vi "sever-client.vi"() -> ()   [LabVIEW 2020]
uses:
  <vilib>/Utility/sysdir.llb/System Directory Type.ctl
panel:
  in  "s 6":bool=TRUE
  in  "s 5":bool
  in  "s 4":bool=TRUE
  in  "批量发送菜单":bool
  out "接收数据":string
  in  "发送数据":string
  out "远程端口":u16
  out "远程地址":string
  in  "批量发送":string[][](table)=[["Date", "Delay(ms)"], ["", ""], ["", ""], ["", ""], ["", ""], ["", ""]]
  in  "定时间隔毫秒":dbl=1000.0
  in  "定时发送":bool
  out "当前发送":string
  out "数值":dbl
  out "times":dbl
  in  "s 3":bool
  out "添加的路径":path
  out "每小时读码次数":dbl
  in  "s 2":bool
  out "时间统计":string
  in  "s":bool
  out "total times":dbl
  out "standard output":string caption="PING标准输出"
  in  "停止":bool
  in  "开启检测模式":bool
  out "误码次数":dbl
  in  "标准码词":string="\r"
  in  "十六进制显示":bool
  in  "自动换行":bool=TRUE
  in  "时间显示":bool=TRUE
  in  "接收超时毫秒":i32=200
  in  "清空接收数据区":bool
  in  "读取的字节":i32=500
  in  "十六进制发送":bool=TRUE
  in  "清空发送数据区":bool
  in  "发送超时毫秒":i32=200
  in  "发送":bool
  in  "数据保存":bool
  in  "路径":path
  in  "服务器IP地址":string="192.168.1.103"
  in  "sever-client":u16(ring) items=["TCP-Sever", "TCP-client"]
  in  "服务器端口号":u16=34567
  in  "开始":bool
  out "错误输出":errorcluster caption="TCP错误输出"
  # "V1.0.1"
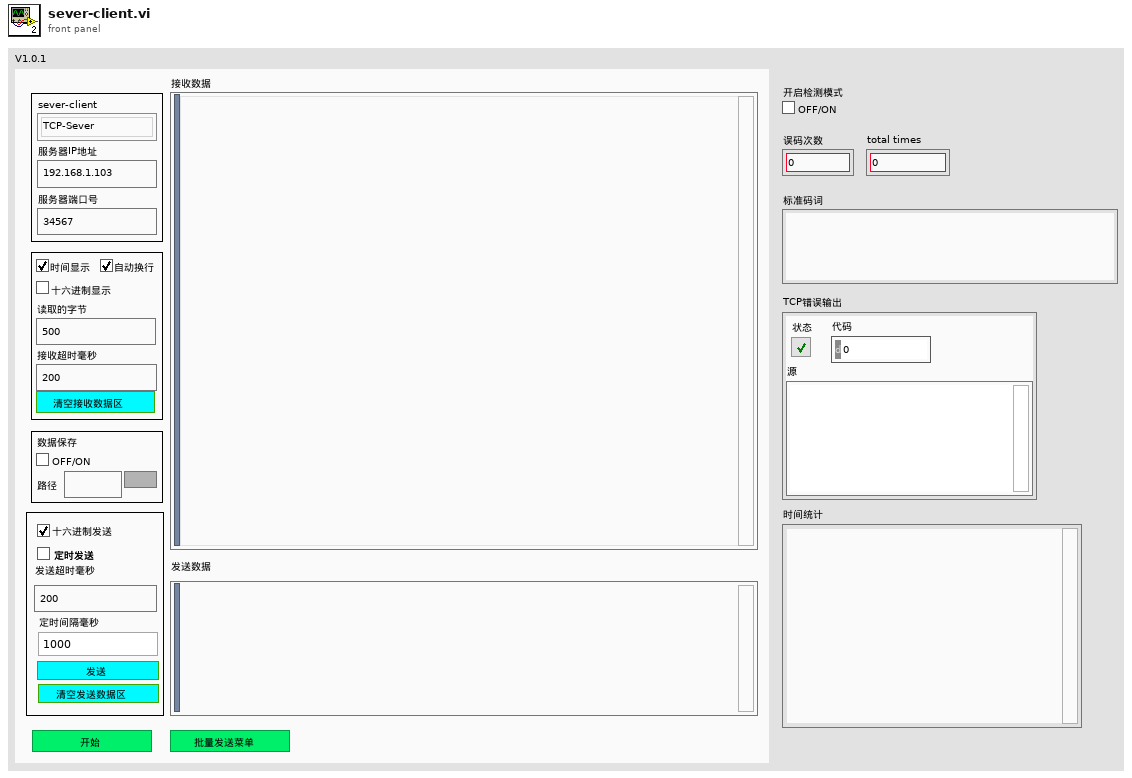
[diagram p1: front panel]
types:
  T1 = typedef "System Directory Type.ctl" = i32
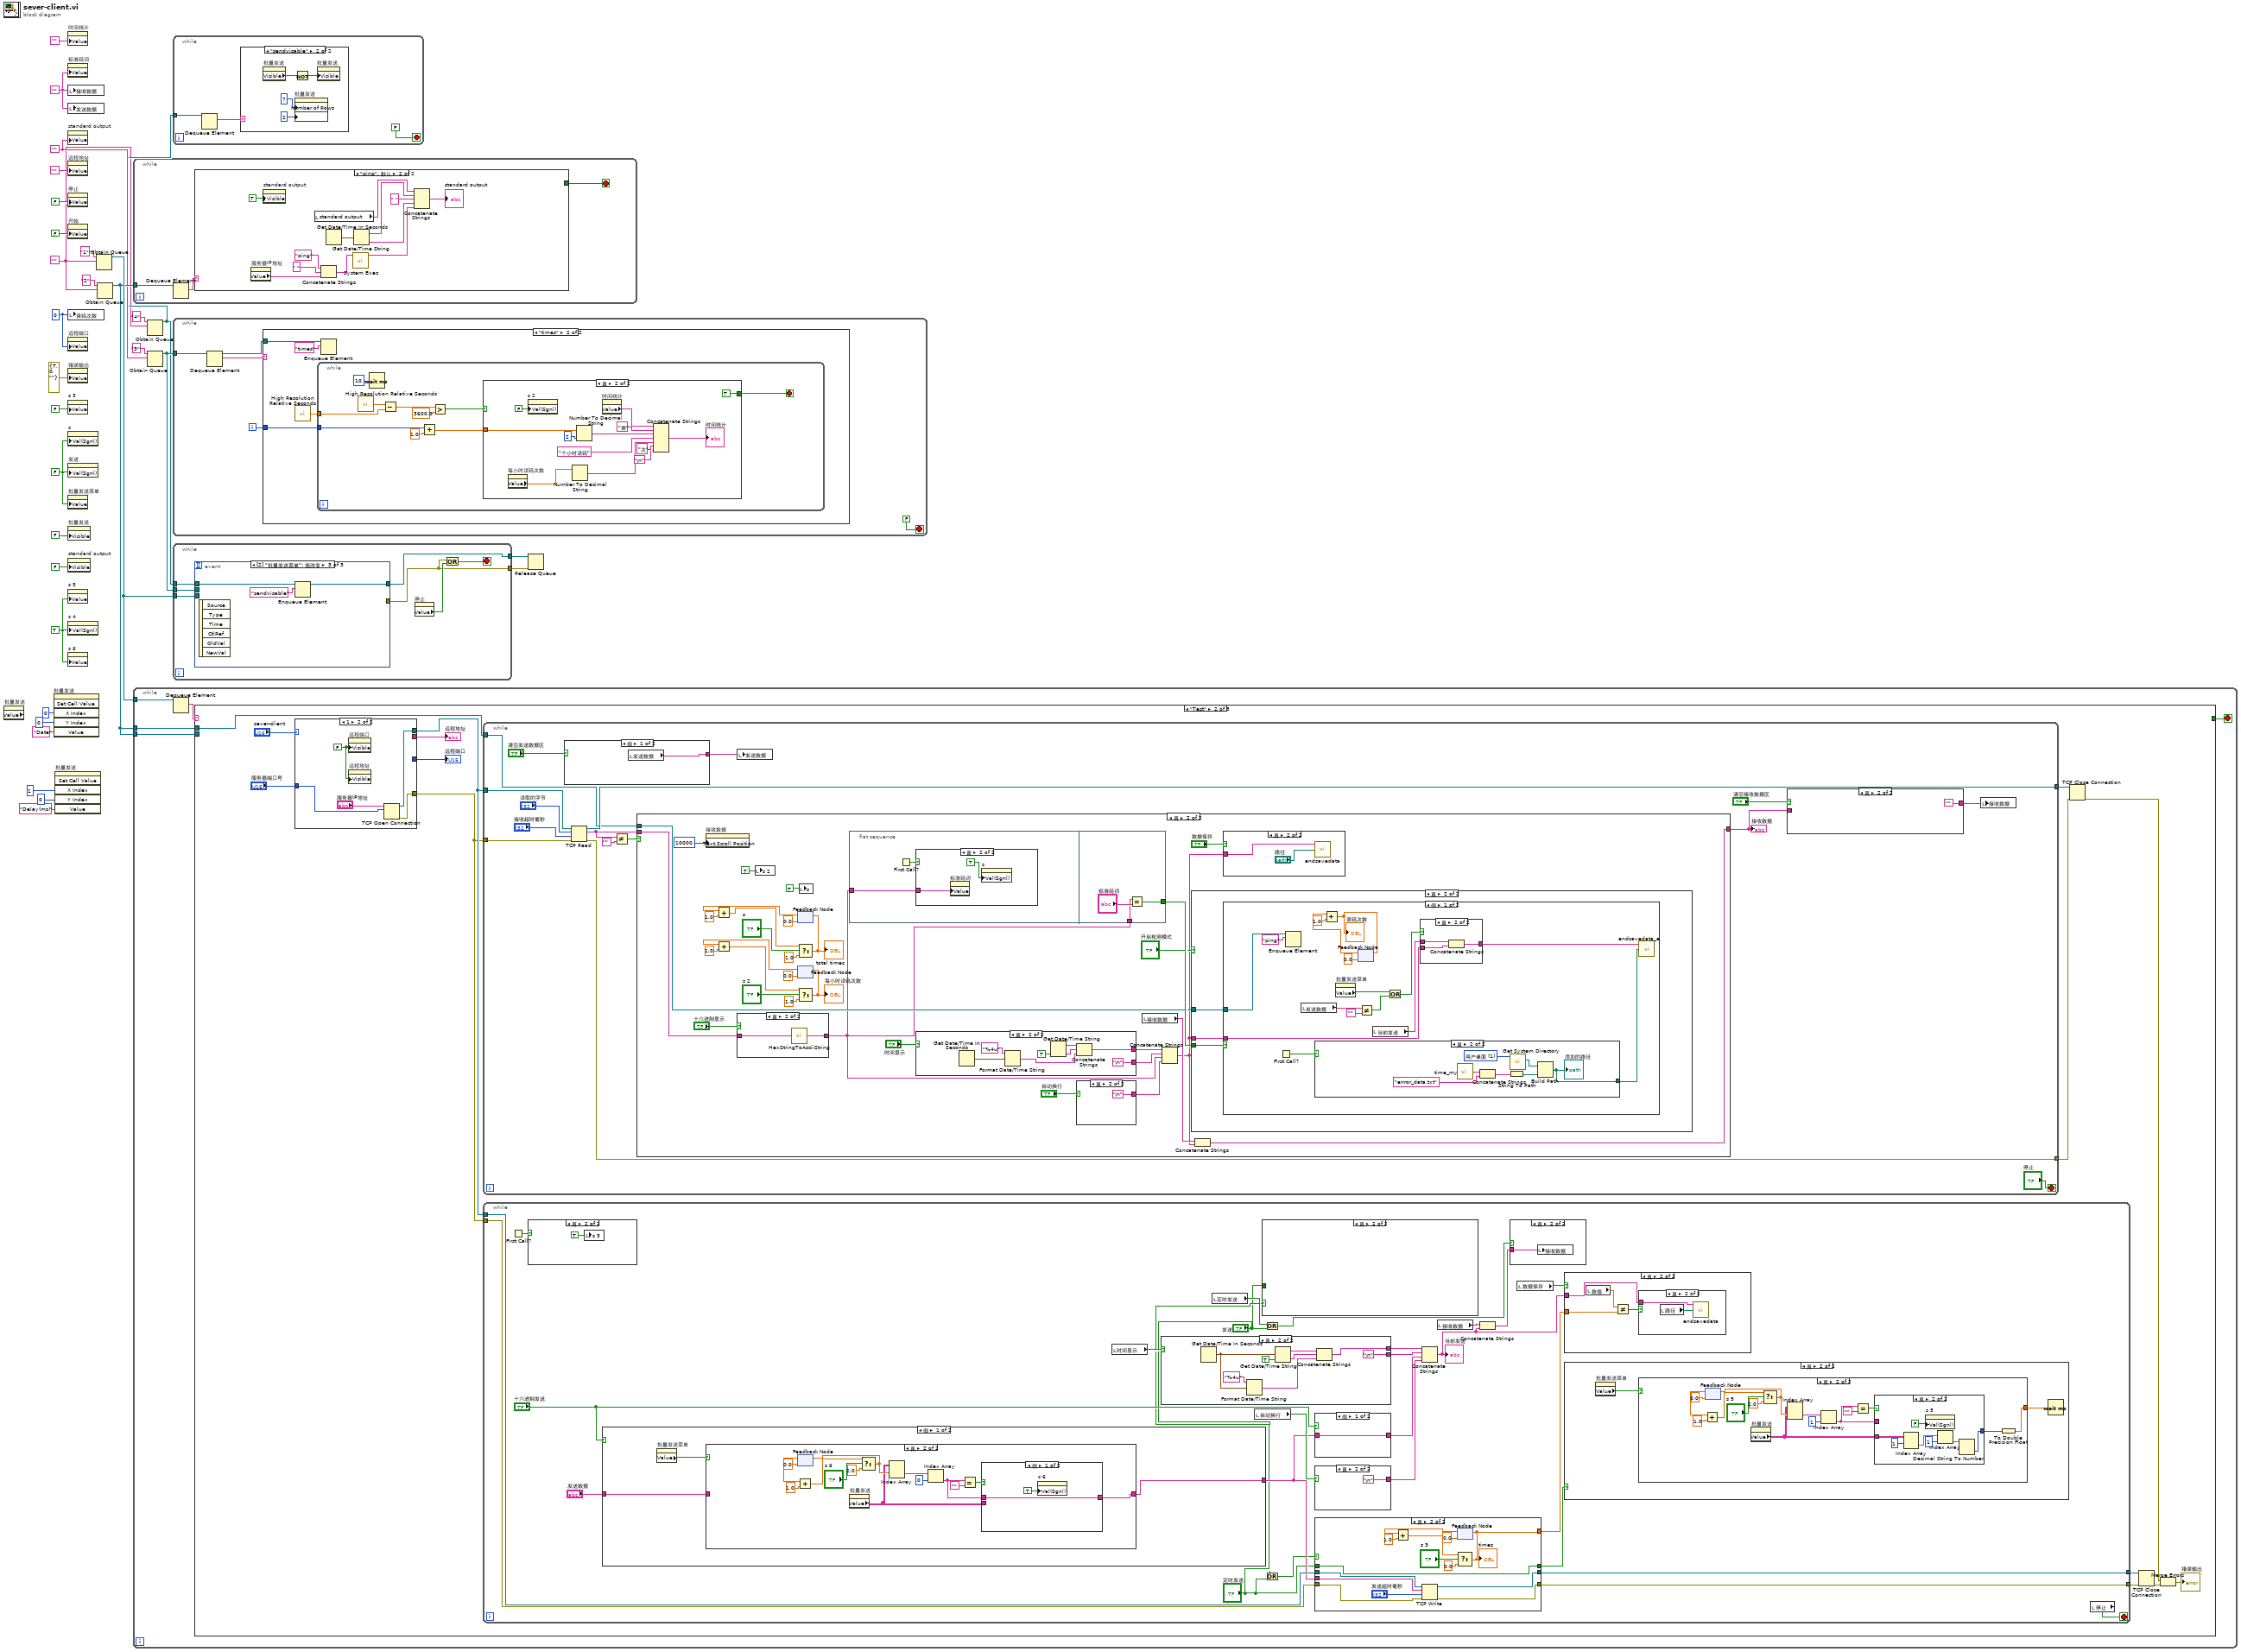
[diagram p0: block diagram]
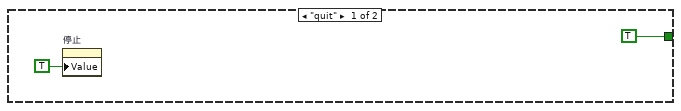
[diagram p5: hidden frame]
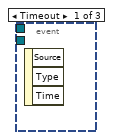
[diagram p6: hidden frame]
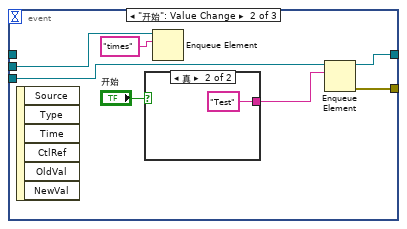
[diagram p7: hidden frame]
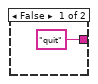
[diagram p8: hidden frame]
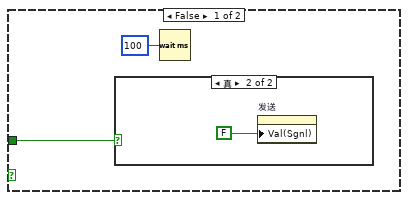
[diagram p10: hidden frame]
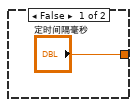
[diagram p13: hidden frame]
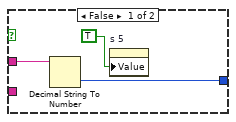
[diagram p14: hidden frame]
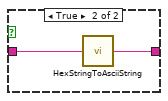
[diagram p17: hidden frame]
diagram:
  w8 = TRUE ("值(信号)")
  w7 = u16 0 ("远程端口")
  w15 = ""
  w10 = FALSE ("值(信号)")
  w18 = ""
  w12 = ""
  n1 = property on="批量发送" class="Tbl (严格)" props=["Value"]() -> ()  [unwired: 2 in, 3 out]
  n2 = invoke on="批量发送" class="Tbl (严格)" method="Set Cell Value"("X Index"=0 ("X索引"), "Y Index"=0 ("Y索引"), "Value"="Date" ("值")) -> ()  [unwired: 3 in, 6 out]
  n3 = invoke on="批量发送" class="Tbl (严格)" method="Set Cell Value"("X Index"=1 ("X索引"), "Y Index"=0 ("Y索引"), "Value"="Delay(ms)" ("值")) -> ()  [unwired: 3 in, 6 out]
  n4 = property on="时间统计" class="Str"("Value"="") -> ()  [unwired: 2 in, 2 out]
  n5 = property on="标准码词" class="Str"("Value"=w15) -> ()  [unwired: 2 in, 2 out]
  n6 = local write "接收数据"(w15) -> ()
  n7 = local write "发送数据"(w15) -> ()
  n8 = property on="standard output" class="Str"("Value"=w18) -> ()  [unwired: 2 in, 2 out]
  n9 = property on="远程地址" class="Str"("Value"="") -> ()  [unwired: 2 in, 2 out]
  n10 = property on="停止" class="Bool (严格)"("Value"=FALSE ("停止")) -> ()  [unwired: 2 in, 2 out]
  n11 = property on="开始" class="Bool (严格)"("Value"=FALSE ("开始")) -> ()  [unwired: 2 in, 2 out]
  n12 = local write "误码次数"(w7) -> ()
  n13 = property on="远程端口" class="DigNum (严格)"("Value"=w7) -> ()  [unwired: 2 in, 2 out]
  n14 = property on="错误输出" class="Clust (严格)"("Value"=errorcluster {"status"=TRUE, "code"=0, "source"=""} ("错误输出")) -> ()  [unwired: 2 in, 2 out]
  n15 = property on="s 3" class="Bool (严格)"("Value"=FALSE ("s 3")) -> ()  [unwired: 2 in, 2 out]
  n16 = property on="s" class="Bool (严格)"("Val(Sgnl)"=w10) -> ()  [unwired: 2 in, 2 out]
  n17 = property on="发送" class="Bool (严格)"("Val(Sgnl)"=w10) -> ()  [unwired: 2 in, 2 out]
  n18 = property on="批量发送菜单" class="Bool (严格)"("Value"=w10) -> ()  [unwired: 2 in, 2 out]
  n19 = property on="批量发送" class="Tbl (严格)"("Visible"=FALSE ("可见")) -> ()  [unwired: 2 in, 2 out]
  n20 = property on="standard output" class="Str"("Visible"=FALSE ("可见")) -> ()  [unwired: 2 in, 2 out]
  n21 = property on="s 5" class="Bool (严格)"("Value"=w8) -> ()  [unwired: 2 in, 2 out]
  n22 = property on="s 4" class="Bool (严格)"("Val(Sgnl)"=w8) -> ()  [unwired: 2 in, 2 out]
  n23 = property on="s 6" class="Bool (严格)"("Value"=w8) -> ()  [unwired: 2 in, 2 out]
  n24 = Obtain Queue(name (unnamed)="1" ("名称（未命名）"), element data type=w12) -> (queue out=w29:refnum<queue>)  [unwired: 3 in, 2 out]
  n25 = Obtain Queue(name (unnamed)="2" ("名称（未命名）"), element data type=w12) -> (queue out=w25:refnum<queue>)  [unwired: 3 in, 2 out]
  n26 = while {
    tunnel: w25 -> [w31]
    stop <- w32 stop-if-true
    n27 = Dequeue Element(queue=w31) -> (element=w33:string)  [unwired: 2 in, 3 out]
    n28 = case shown="\"ping\", 默认" w33 {
      tunnel: [TRUE _] -> w32
      frame "quit" {
        n29 = property on="停止" class="Bool (严格)"("Value"=TRUE ("停止")) -> ()  [unwired: 2 in, 2 out]
      }
      frame "ping", Default {
        n30 = property on="服务器IP地址" class="Str"() -> ("Value"=w45:string)  [unwired: 2 in, 2 out]
        n31 = property on="standard output" class="Str"("Visible"=TRUE ("可见")) -> ()  [unwired: 2 in, 2 out]
        n32 = local read "standard output"() -> (w37:string)
        n33 = Concatenate Strings("ping" ("字符串"), " " ("字符串"), w45) -> (w44:string)
        n34 = Get Date/Time In Seconds() -> (seconds since 1Jan1904=w42:timestamp)
        n35 = call <vilib>:"System Exec.vi"("command line"=w44) -> ("standard output"=w43:string)  [unwired: 7 in, 3 out]
        n36 = Get Date/Time String(seconds (now)=w42) -> (date string=w41:string, time string=w39:string)  [unwired: 2 in]
        n37 = Concatenate Strings(w37, w41, " " ("字符串"), w39, w43) -> (→"standard output":string)
      }
    }
  }
  n38 = while {
    tunnel: w29 -> [w50]
    tunnel: w25 -> [w49]
    tunnel: w25 -> [w48]
    stop <- w52 stop-if-true
    n39 = Dequeue Element(queue=w50) -> (element=w51:string)  [unwired: 2 in, 3 out]
    n40 = case shown="\"Test\"" w51 {
      tunnel: [_ _ TRUE] -> w52
      tunnel: w49 -> [_ w61 _]
      tunnel: w48 -> [_ _ w342]
      frame "假", Default {
      }
      frame "Test" {
        n41 = case shown="1" "sever-client" {
          tunnel: "服务器端口号" -> [w226 w231]
          tunnel: [w225 w230] -> w60
          tunnel: [w224 w229] -> w59
          tunnel: [w223 _] -> w64
          tunnel: [w222 _] -> w63
          frame 0, Default {
            w221 = TRUE
            n42 = property on="远程端口" class="DigNum (严格)"("Visible"=w221) -> ()  [unwired: 2 in, 2 out]
            n43 = property on="远程地址" class="Str"("Visible"=w221) -> ()  [unwired: 2 in, 2 out]
            n44 = call <vilib>:"TCP Listen.vi"("port"=w226) -> ("error out"=w224:errorcluster, "remote port"=w222:u16, "remote address"=w223:string, "connection ID"=w225:refnum<k5>)  [unwired: 6 in, 1 out]
          }
          frame 1 {
            w227 = FALSE
            n45 = property on="远程端口" class="DigNum (严格)"("Visible"=w227) -> ()  [unwired: 2 in, 2 out]
            n46 = property on="远程地址" class="Str"("Visible"=w227) -> ()  [unwired: 2 in, 2 out]
            n47 = TCP Open Connection(address="服务器IP地址", remote port or service name=w231) -> (connection ID=w230:refnum<k5>, error out=w229:errorcluster)  [unwired: 3 in]
          }
        }
        "远程地址" <- w64
        "远程端口" <- w63
        n48 = while {
          tunnel: [w245] -> w54
          tunnel: [w237] -> w62
          tunnel: w61 -> [w236]
          tunnel: w60 -> [w234]
          tunnel: w59 -> [w233]
          stop <- "停止" stop-if-true
          n49 = case shown="假" "清空发送数据区" {
            tunnel: [w248 ""] -> w238
            frame False {
              n50 = local read "发送数据"() -> (w248:string)
            }
            frame True {
            }
          }
          n51 = TCP Read(connection ID=w234, bytes to read="读取的字节", error in (no error)=w233, 9:"接收超时毫秒") -> (connection ID out=w245:refnum<k5>, data out=w243:string, error out=w237:errorcluster)  [unwired: 1 in]
          n52 = Not Equal?(x=w243, y="") -> (x != y?=w232:bool)
          n53 = case shown="真" w232 {
            tunnel: w243 -> [_ w284]
            tunnel: [w257 w286] -> w240
            tunnel: w236 -> [_ w280]
            frame False {
              n54 = local read "接收数据"() -> (w257:string)
            }
            frame True {
              n55 = property on="接收数据" class="Str"("Text.Scroll Position"=u32 10000 ("文本.滚动条位置")) -> ()  [unwired: 2 in, 2 out]
              n56 = case shown="真" "十六进制显示" {
                tunnel: [w328 w330] -> w262
                tunnel: w284 -> [w328 w329]
                frame False {
                }
                frame True {
                  n57 = call "HexStringToAsciiString.vi"("输入Hex字符串"=w329) -> ("输出Ascii"=w330:string)
                }
              }
              n58 = local write "s 2"(TRUE ("值(信号)")) -> ()
              n59 = feedback #1(0.0 ("x")) -> (w276:dbl)
              n60 = Add(x=w276, y=1.0) -> (x+y=w275:dbl)
              n61 = Select(t=w275, s="s", f=1.0) -> (s? t:f=w272:dbl)
              "total times" <- w272
              n62 = feedback-in #1(w272) -> ()
              n63 = feedback #2(0.0 ("x")) -> (w269:dbl)
              n64 = Add(x=w269, y=1.0) -> (x+y=w270:dbl)
              n65 = Select(t=w270, s="s 2", f=1.0) -> (s? t:f=w265:dbl)
              "每小时读码次数" <- w265
              n66 = feedback-in #2(w265) -> ()
              n67 = local write "s"(TRUE ("值(信号)")) -> ()
              n68 = flat-sequence {
                tunnel: w262 -> [w290]
                tunnel: w262 -> [w294]
                tunnel: [w295] -> w283
                frame #0 {
                  n69 = First Call?() -> (First Call?: T/F=w291:bool)
                  n70 = case shown="真" w291 {
                    tunnel: w290 -> [_ w293]
                    frame False {
                    }
                    frame True {
                      n71 = property on="标准码词" class="Str"("Value"=w293) -> ()  [unwired: 2 in, 2 out]
                      n72 = property on="s" class="Bool (严格)"("Val(Sgnl)"=TRUE ("值(信号)")) -> ()  [unwired: 2 in, 2 out]
                    }
                  }
                }
                frame #1 {
                  n73 = Equal?(x=w294, y="标准码词") -> (x = y?=w295:bool)
                }
              }
              n74 = case shown="真" "时间显示" {
                tunnel: [_ w338] -> w264
                tunnel: [_ "\n"] -> w263
                frame False {
                }
                frame True {
                  n75 = Get Date/Time In Seconds() -> (seconds since 1Jan1904=w335:timestamp)
                  n76 = Format Date/Time String(time format string (%c)="%4u" ("时间格式字符串(%c)"), seconds (now)=w335) -> (date/time string=w334:string)  [unwired: 1 in]
                  n77 = Get Date/Time String(want seconds? (F)=TRUE ("需要秒？(F)")) -> (date string=w340:string, time string=w339:string)  [unwired: 2 in]
                  n78 = Concatenate Strings(w340, w339, w334) -> (w338:string)
                }
              }
              n79 = case shown="真" "自动换行" {
                tunnel: [_ "\n"] -> w261
                frame False {
                }
                frame True {
                }
              }
              n80 = local read "接收数据"() -> (w288:string)
              n81 = Concatenate Strings(w264, w263, w262, w261) -> (w260:string)
              n82 = case shown="真" "开启检测模式" {
                tunnel: w283 -> [_ w299]
                tunnel: w280 -> [_ w298]
                tunnel: w260 -> [_ w297]
                frame False {
                }
                frame True {
                  n83 = case shown="假" w299 {
                    tunnel: w298 -> [w310 _]
                    tunnel: w297 -> [w306 _]
                    frame False {
                      n84 = First Call?() -> (First Call?: T/F=w309:bool)
                      n85 = Enqueue Element(queue=w310, element="ping" ("元素")) -> ()  [unwired: 2 in, 3 out]
                      n86 = local read "发送数据"() -> (w304:string)
                      n87 = case shown="真" w309 {
                        tunnel: [w320 w323] -> w308
                        frame False {
                          n88 = local read "添加的路径"() -> (w320:path)
                        }
                        frame True {
                          w327 = T1 1 items=["用户目录"=0, "用户桌面"=1, "用户文档"=2, "用户应用程序数据"=3, "用户设置"=4, "用户临时目录"=5, "公共文档"=6, "公共应用程序数据"=7, "公共设置"=8, "公共缓存"=13, "系统核心库"=9, "系统安装库"=10, "应用程序文件"=11, "启动盘根目录"=12] ("system directory type")
                          n89 = call "time_my.vi"() -> ("时间"=w321:string)
                          n90 = Concatenate Strings(w321, "errror_data.txt") -> (w325:string)
                          n91 = String To Path(string=w325) -> (path=w324:path)
                          n92 = call <vilib>:"Get System Directory.vi"("system directory type"=w327) -> ("system directory"=w326:path)  [unwired: 10 in]
                          n93 = Build Path(base path=w326, name or relative path=w324) -> (appended path=w323:path)
                          "添加的路径" <- w323
                        }
                      }
                      n94 = property on="批量发送菜单" class="Bool (严格)"() -> ("Value"=w302:bool)  [unwired: 2 in, 2 out]
                      n95 = feedback #3(0.0) -> (w312:dbl)
                      n96 = Add(x=w312, y=1.0) -> (x+y=w314:dbl)
                      "误码次数" <- w314
                      n97 = feedback-in #3(w314) -> ()
                      n98 = Not Equal?(x=w304, y="") -> (x != y?=w303:bool)
                      n99 = local read "当前发送"() -> (w305:string)
                      n100 = Or(x=w302, y=w303) -> (x .or. y?=w301:bool)
                      n101 = case shown="真" w301 {
                        tunnel: [w316 w317] -> w307
                        tunnel: w306 -> [w316 w318]
                        tunnel: w305 -> [_ w319]
                        frame False {
                        }
                        frame True {
                          n102 = Concatenate Strings(w319, w318) -> (w317:string)
                        }
                      }
                      n103 = call "endsavedata_e.vi"("文件路径（使用对话框）"=w308, "文本"=w307) -> ()  [unwired: 1 in, 2 out]
                    }
                    frame True {
                    }
                  }
                }
              }
              n104 = Concatenate Strings(w288, w260) -> (w286:string)
              n105 = case shown="真" "数据保存" {
                tunnel: w260 -> [_ w331]
                frame False {
                }
                frame True {
                  n106 = call "endsavedata.vi"("文件路径（使用对话框）"="路径", "文本"=w331) -> ()  [unwired: 1 in, 2 out]
                }
              }
            }
          }
          "接收数据" <- w240
          n107 = local write "发送数据"(w238) -> ()
          n108 = case shown="真" "清空接收数据区" {
            tunnel: [w253 ""] -> w242
            tunnel: w240 -> [w251 _]
            frame False {
              n109 = String Length(string=w251) -> (length=w255:i32)
              n110 = Greater?(x=w255, y=10000) -> (0:w254:bool)
              n111 = Select(t="", s=w254, f=w251) -> (s? t:f=w253:string)
            }
            frame True {
            }
          }
          n112 = local write "接收数据"(w242) -> ()
        }
        n113 = while {
          tunnel: w60 -> [w92]
          tunnel: w59 -> [w91]
          tunnel: [w90] -> w58
          tunnel: [w73] -> w53
          stop <- w89 stop-if-true
          n114 = First Call?() -> (First Call?: T/F=w77:bool)
          n115 = case shown="真" w77 {
            frame False {
            }
            frame True {
              n116 = local write "s 3"(TRUE ("s 3")) -> ()
            }
          }
          n117 = case shown="假" "十六进制发送" {
            selector: "十六进制发送" -> [_ w181]
            tunnel: "发送数据" -> [w157 w184]
            tunnel: [w156 w183] -> w82
            frame False {
              n118 = property on="批量发送菜单" class="Bool (严格)"() -> ("Value"=w155:bool)  [unwired: 2 in, 2 out]
              n119 = case shown="真" w155 {
                tunnel: [w158 w161] -> w156
                tunnel: w157 -> [w158 _]
                frame False {
                }
                frame True {
                  n120 = feedback #4(0.0 ("x")) -> (w169:dbl)
                  n121 = Add(x=w169, y=1.0) -> (x+y=w166:dbl)
                  n122 = property on="批量发送" class="Tbl (严格)"() -> ("Value"=w159:string[][])  [unwired: 2 in, 2 out]
                  n123 = Select(t=w166, s="s 6", f=2.0) -> (s? t:f=w165:dbl)
                  n124 = feedback-in #4(w165) -> ()
                  n125 = Index Array(array=w159, index (row)=w165) -> (element=w172:string[])  [unwired: 1 in]
                  n126 = Index Array(array=w172, index=0 ("索引")) -> (element=w160:string)
                  n127 = Equal?(x=w160, y="") -> (x = y?=w162:bool)
                  n128 = case shown="假" w162 {
                    tunnel: [w174 w178] -> w161
                    tunnel: w160 -> [w174 _]
                    tunnel: w159 -> [_ w180]
                    frame False {
                      n129 = property on="s 6" class="Bool (严格)"("Val(Sgnl)"=TRUE ("值(信号)")) -> ()  [unwired: 2 in, 2 out]
                    }
                    frame True {
                      n130 = Index Array(array=w180, index (row)=1 ("索引 (行)")) -> (element=w179:string[])  [unwired: 1 in]
                      n131 = property on="s 6" class="Bool (严格)"("Val(Sgnl)"=FALSE ("值(信号)")) -> ()  [unwired: 2 in, 2 out]
                      n132 = Index Array(array=w179, index=0 ("索引")) -> (element=w178:string)
                    }
                  }
                }
              }
            }
            frame True {
              n133 = local read "times"() -> (→"数值":dbl)
              n134 = case shown="真" "批量发送菜单" {
                tunnel: w184 -> [w187 _]
                tunnel: [w186 w198] -> w183
                tunnel: w181 -> [_ w197]
                frame False {
                  n135 = call "AsciiStringToHexString.vi"("输入Asciistring1"=w187) -> ("输出HexString"=w186:string)
                }
                frame True {
                  n136 = feedback #5(0.0 ("x")) -> (w200:dbl)
                  n137 = Add(x=w200, y=1.0) -> (x+y=w195:dbl)
                  n138 = Select(t=w195, s="s 4", f=2.0) -> (s? t:f=w194:dbl)
                  n139 = feedback-in #5(w194) -> ()
                  n140 = Index Array(array="批量发送", index (row)=w194) -> (element=w203:string[])  [unwired: 1 in]
                  n141 = Index Array(array=w203, index=0 ("索引")) -> (element=w189:string)
                  n142 = Equal?(x=w189, y="") -> (x = y?=w191:bool)
                  n143 = case shown="假" w191 {
                    tunnel: [w205 w209] -> w190
                    tunnel: w189 -> [w205 _]
                    tunnel: "批量发送" -> [_ w211]
                    frame False {
                      n144 = property on="s 4" class="Bool (严格)"("Val(Sgnl)"=TRUE ("值(信号)")) -> ()  [unwired: 2 in, 2 out]
                    }
                    frame True {
                      n145 = Index Array(array=w211, index (row)=1 ("索引 (行)")) -> (element=w210:string[])  [unwired: 1 in]
                      n146 = property on="s 4" class="Bool (严格)"("Val(Sgnl)"=FALSE ("值(信号)")) -> ()  [unwired: 2 in, 2 out]
                      n147 = Index Array(array=w210, index=0 ("索引")) -> (element=w209:string)
                    }
                  }
                  n148 = case shown="真" w197 {
                    tunnel: [w212 w214] -> w198
                    tunnel: w190 -> [w212 w213]
                    frame False {
                    }
                    frame True {
                      n149 = call "AsciiStringToHexString.vi"("输入Asciistring1"=w213) -> ("输出HexString"=w214:string)
                    }
                  }
                }
              }
            }
          }
          n150 = local read "时间显示"() -> (w74:bool)
          n151 = case shown="真" w74 {
            tunnel: [_ w135] -> w86
            tunnel: [_ "\n"] -> w85
            frame False {
            }
            frame True {
              n152 = Get Date/Time In Seconds() -> (seconds since 1Jan1904=w131:timestamp)
              n153 = Format Date/Time String(time format string (%c)="%4u" ("时间格式字符串(%c)"), seconds (now)=w131) -> (date/time string=w132:string)  [unwired: 1 in]
              n154 = Get Date/Time String(seconds (now)=w131, want seconds? (F)=TRUE ("需要秒？(F)")) -> (date string=w136:string, time string=w133:string)  [unwired: 1 in]
              n155 = Concatenate Strings(w136, w133, w132) -> (w135:string)
            }
          }
          n156 = local read "定时发送"() -> (w72:bool)
          n157 = local read "自动换行"() -> (w87:bool)
          n158 = case shown="真" "定时发送" {
            tunnel: "发送" -> [w94 _]
            frame False {
              n159 = case shown="真" w94 {
                frame False {
                }
                frame True {
                  n160 = property on="发送" class="Bool (严格)"("Val(Sgnl)"=FALSE ("值(信号)")) -> ()  [unwired: 2 in, 2 out]
                }
              }
              n161 = Wait (ms)(milliseconds to wait=u32 100 ("等待时间（毫秒）")) -> ()  [unwired: 1 out]
            }
            frame True {
            }
          }
          n162 = Or(x=w72, y="发送") -> (x .or. y?=w71:bool)
          n163 = Or(x="发送", y="定时发送") -> (x .or. y?=w70:bool)
          n164 = case shown="假" "十六进制发送" {
            tunnel: [w126 w128] -> w81
            tunnel: w82 -> [w126 w127]
            frame False {
            }
            frame True {
              n165 = call "HexStringToAsciiString.vi"("输入Hex字符串"=w127) -> ("输出Ascii"=w128:string)
            }
          }
          n166 = case shown="真" w87 {
            tunnel: [_ "\n"] -> w83
            frame False {
            }
            frame True {
            }
          }
          n167 = case shown="真" w70 {
            tunnel: w82 -> [_ w150]
            tunnel: [w140 w154] -> w73
            tunnel: [w139 w153] -> w90
            tunnel: w92 -> [w140 w152]
            tunnel: w91 -> [w139 w151]
            tunnel: [_ w143] -> w76
            tunnel: "定时发送" -> [w138 w142]
            tunnel: [w138 w142] -> w69
            frame False {
            }
            frame True {
              n168 = TCP Write(connection ID=w152, data in=w150, error in (no error)=w151, 9:"发送超时毫秒") -> (connection ID out=w154:refnum<k5>, error out=w153:errorcluster)  [unwired: 1 out]
              n169 = feedback #6(0.0 ("x")) -> (w144:dbl)
              n170 = Add(x=w144, y=1.0) -> (x+y=w149:dbl)
              n171 = Select(t=w149, s="s 3", f=0.0) -> (s? t:f=w143:dbl)
              "times" <- w143
              n172 = feedback-in #6(w143) -> ()
            }
          }
          n173 = Concatenate Strings(w86, w85, w81, w83) -> (w79:string)
          "当前发送" <- w79
          n174 = local read "接收数据"() -> (w84:string)
          n175 = Concatenate Strings(w84, w79) -> (w78:string)
          n176 = case shown="真" w71 {
            tunnel: w78 -> [_ w125]
            frame False {
            }
            frame True {
              n177 = local write "接收数据"(w125) -> ()
            }
          }
          n178 = local read "数据保存"() -> (w75:bool)
          n179 = case shown="真" w75 {
            tunnel: w79 -> [_ w218]
            tunnel: w76 -> [_ w216]
            frame False {
            }
            frame True {
              n180 = local read "数值"() -> (w215:dbl)
              n181 = Not Equal?(x=w215, y=w216) -> (x != y?=w217:bool)
              n182 = case shown="真" w217 {
                tunnel: w218 -> [_ w219]
                frame False {
                }
                frame True {
                  n183 = local read "路径"() -> (w220:path)
                  n184 = call "endsavedata.vi"("文件路径（使用对话框）"=w220, "文本"=w219) -> ()  [unwired: 1 in, 2 out]
                }
              }
            }
          }
          n185 = case shown="真" w69 {
            frame False {
            }
            frame True {
              n186 = property on="批量发送菜单" class="Bool (严格)"() -> ("Value"=w96:bool)  [unwired: 2 in, 2 out]
              n187 = case shown="真" w96 {
                tunnel: ["定时间隔毫秒" w99] -> w97
                frame False {
                }
                frame True {
                  n188 = feedback #7(0.0 ("x")) -> (w109:dbl)
                  n189 = Add(x=w109, y=1.0) -> (x+y=w108:dbl)
                  n190 = property on="批量发送" class="Tbl (严格)"() -> ("Value"=w103:string[][])  [unwired: 2 in, 2 out]
                  n191 = Select(t=w108, s="s 5", f=2.0) -> (s? t:f=w104:dbl)
                  n192 = feedback-in #7(w104) -> ()
                  n193 = Index Array(array=w103, index (row)=w104) -> (element=w113:string[])  [unwired: 1 in]
                  n194 = Index Array(array=w113, index=1 ("索引")) -> (element=w107:string)
                  n195 = Equal?(x=w107, y="") -> (x = y?=w105:bool)
                  n196 = case shown="真" w105 {
                    tunnel: w107 -> [w116 _]
                    tunnel: [w115 w118] -> w100
                    tunnel: w103 -> [_ w122]
                    frame False {
                      n197 = Decimal String To Number(string=w116) -> (number=w115:i32)  [unwired: 2 in, 1 out]
                      n198 = property on="s 5" class="Bool (严格)"("Value"=TRUE ("s 5")) -> ()  [unwired: 2 in, 2 out]
                    }
                    frame True {
                      n199 = Index Array(array=w122, index (row)=1 ("索引 (行)")) -> (element=w121:string[])  [unwired: 1 in]
                      n200 = property on="s 5" class="Bool (严格)"("Val(Sgnl)"=FALSE ("值(信号)")) -> ()  [unwired: 2 in, 2 out]
                      n201 = Index Array(array=w121, index=1 ("索引")) -> (element=w119:string)
                      n202 = Decimal String To Number(string=w119) -> (number=w118:i32)  [unwired: 2 in, 1 out]
                    }
                  }
                  n203 = To Double Precision Float(number=w100) -> (double precision float=w99:dbl)
                }
              }
              n204 = Wait (ms)(milliseconds to wait=w97) -> ()  [unwired: 1 out]
            }
          }
          n205 = local read "停止"() -> (w89:bool)
        }
        n206 = TCP Close Connection(connection ID=w54, error in (no error)=w62) -> (error out=w56:errorcluster)  [unwired: 1 in, 1 out]
        n207 = TCP Close Connection(connection ID=w53, error in (no error)=w58) -> (error out=w57:errorcluster)  [unwired: 1 in, 1 out]
        n208 = Merge Errors(w56, w57) -> (→"错误输出":errorcluster)
      }
      frame "quit" {
        n209 = Enqueue Element(queue=w342, element="quit" ("元素")) -> ()  [unwired: 2 in, 3 out]
      }
    }
  }
  n210 = Obtain Queue(name (unnamed)="4" ("名称（未命名）"), element data type=w12) -> (queue out=w13:refnum<queue>)  [unwired: 3 in, 2 out]
  n211 = Obtain Queue(name (unnamed)="3" ("名称（未命名）"), element data type=w18) -> (queue out=w20:refnum<queue>)  [unwired: 3 in, 2 out]
  n212 = while {
    tunnel: w13 -> [w346]
    stop <- FALSE stop-if-true
    n213 = Dequeue Element(queue=w346) -> (element=w347:string)  [unwired: 2 in, 3 out]
    n214 = case shown="\"sendvisable\"" w347 {
      frame "假", Default {
      }
      frame "sendvisable" {
        n215 = property on="批量发送" class="Tbl (严格)"() -> ("Visible"=w351:bool)  [unwired: 2 in, 2 out]
        n216 = Not(x=w351) -> (.not. x?=w350:bool)
        n217 = property on="批量发送" class="Tbl (严格)"("Number of Rows"=u32 7 ("行数"), "Number of Columns"=u32 2 ("列数")) -> ()  [unwired: 2 in, 2 out]
        n218 = property on="批量发送" class="Tbl (严格)"("Visible"=w350) -> ()  [unwired: 2 in, 2 out]
      }
    }
  }
  n219 = while {
    tunnel: w20 -> [w354]
    i -> [w353]
    stop <- FALSE stop-if-true
    n220 = Dequeue Element(queue=w354) -> (queue out=w352:refnum<queue>, element=w355:string)  [unwired: 2 in, 2 out]
    n221 = case shown="\"times\"" w355 {
      tunnel: w353 -> [_ w359]
      tunnel: w352 -> [_ w358]
      frame "假", Default {
      }
      frame "times" {
        n222 = call <vilib>:"High Resolution Relative Seconds.vi"() -> ("relative seconds"=w360:dbl)
        n223 = while {
          tunnel: w360 -> [w369]
          tunnel: w359 -> [w362]
          stop <- w365 stop-if-true
          n224 = call <vilib>:"High Resolution Relative Seconds.vi"() -> ("relative seconds"=w370:dbl)
          n225 = Wait (ms)(milliseconds to wait=u32 10 ("等待时间（毫秒）")) -> ()  [unwired: 1 out]
          n226 = Subtract(x=w370, y=w369) -> (x-y=w368:dbl)
          n227 = Add(x=w362, y=1.0) -> (x+y=w361:dbl)
          n228 = Greater?(x=w368, y=3600.0) -> (0:w366:bool)
          n229 = case shown="真" w366 {
            tunnel: [_ TRUE] -> w365
            tunnel: w361 -> [_ w378]
            frame False {
            }
            frame True {
              n230 = property on="每小时读码次数" class="DigNum (严格)"() -> ("Value"=w375:dbl)  [unwired: 2 in, 2 out]
              n231 = property on="s 2" class="Bool (严格)"("Val(Sgnl)"=FALSE ("s 2")) -> ()  [unwired: 2 in, 2 out]
              n232 = Number To Decimal String(number=w375) -> (decimal integer string=w374:string)  [unwired: 1 in]
              n233 = Number To Decimal String(number=w378, width (-)=i16 2 ("宽度(-)")) -> (decimal integer string=w377:string)
              n234 = property on="时间统计" class="Str"() -> ("Value"=w373:string)  [unwired: 2 in, 2 out]
              n235 = Concatenate Strings(w373, "第" ("字符串"), w377, "个小时读码" ("字符串"), w374, "次" ("字符串"), "\n") -> (→"时间统计":string)
            }
          }
        }
        n236 = Enqueue Element(queue=w358, element="times" ("元素")) -> ()  [unwired: 2 in, 3 out]
      }
    }
  }
  n237 = while {
    tunnel: w29 -> [w390]
    tunnel: [w387] -> w28
    tunnel: [w386] -> w27
    tunnel: w20 -> [w385]
    tunnel: w13 -> [w384]
    stop <- w388 stop-if-true
    n238 = event shown="[2] \"批量发送菜单\": 值改变" {
      selector: _ -> [_ _ _]
      dyn-events: _ -> [_ _ _]
      timeout: _ -> [_ _ _]
      tunnel: w390 -> [_ w397 _]
      tunnel: [_ w394 _] -> w386
      tunnel: [_ w393 w400] -> w387
      tunnel: w385 -> [_ w392 _]
      tunnel: w384 -> [_ _ w402]
      event Timeout {
        n239 = event-data() -> ()  [unwired: 1 in, 3 out]
      }
      event "开始": Value Change {
        n240 = event-data() -> ()  [unwired: 1 in, 6 out]
        n241 = case shown="真" "开始" {
          tunnel: ["quit" ("元素") "Test" ("元素")] -> w395
          frame False {
          }
          frame True {
          }
        }
        n242 = Enqueue Element(queue=w392, element="times" ("元素")) -> ()  [unwired: 2 in, 3 out]
        n243 = Enqueue Element(queue=w397, element=w395) -> (queue out=w393:refnum<queue>, error out=w394:errorcluster)  [unwired: 2 in, 1 out]
      }
      event "批量发送菜单": Value Change {
        n244 = event-data() -> ()  [unwired: 1 in, 6 out]
        n245 = Enqueue Element(queue=w402, element="sendvisable" ("元素")) -> (queue out=w400:refnum<queue>)  [unwired: 2 in, 2 out]
      }
    }
    n246 = property on="停止" class="Bool (严格)"() -> ("Value"=w389:bool)  [unwired: 2 in, 2 out]
    n247 = Or(x=w386, y=w389) -> (x .or. y?=w388:bool)
  }
  n248 = Release Queue(queue=w28, error in (no error)=w27) -> ()  [unwired: 1 in, 3 out]
